vi "setting.vi"(8 "error in (no error)":errorcluster caption="错误输入（无错误）") -> (0 "error out":errorcluster caption="错误输出", 3 "设置":T1)   [LabVIEW 2018]
panel:
  in  "采集设置":T2={"Resource Name"="DAQ::1", "Input Impedance"=0, "采集通道"=2, "Trigger Level (V)"=0.5, "Coupling"=1, "Trigger Slope"=0, "Min Record Length"=40000, "Min. Sample Rate"=10000000.0, "Vertical Range (V)"=5.0, "触发通道"=2} {"触发通道" items=["ch0", "ch1", "ch2", "ch3", "ch4", "ch5", "ch6", "ch7"]; "Vertical Range (V)" format="%_3g"; "Min. Sample Rate" min=10.0 max=60000000.0 format="%#_6p"; "Trigger Slope" items=["Positive", "Negative"]; "Coupling" items=["AC"=0, "DC"=1, "HF Reject"=3, "LF Reject"=4, "AC Plus HF Reject"=1001]; "Trigger Level (V)" format="%.2f"; "采集通道" items=["ch0", "ch1", "ch2", "ch3", "ch4", "ch5", "ch6", "ch7"]; "Input Impedance" items=["1 mega ohm"=0, "50 ohms"=2]}
  in  "矩阵卡设置":cluster{"BUS":u32, "slot":u32}={"BUS"=5, "slot"=5}
  in  "取消按钮":bool
  in  "保存按钮":bool
  in  "模式一设置":T3={"M1-drive-start"=5, "M1-drive-num"=5, "M1-receive-start"=5, "M1-receive-num"=5, "M1-start-delay"=5, "M1-receive-delay"=5}
  in  "模式二设置":T4={"M2-drive-start"=5, "M2-receive-start"=5, "M2-receive-num"=5, "M2-start-delay"=5, "M2-receive-delay"=5}
  # "参数设置"
  # "数据采集"
  # "矩阵开关"
  # "模式一"
  # "模式二"
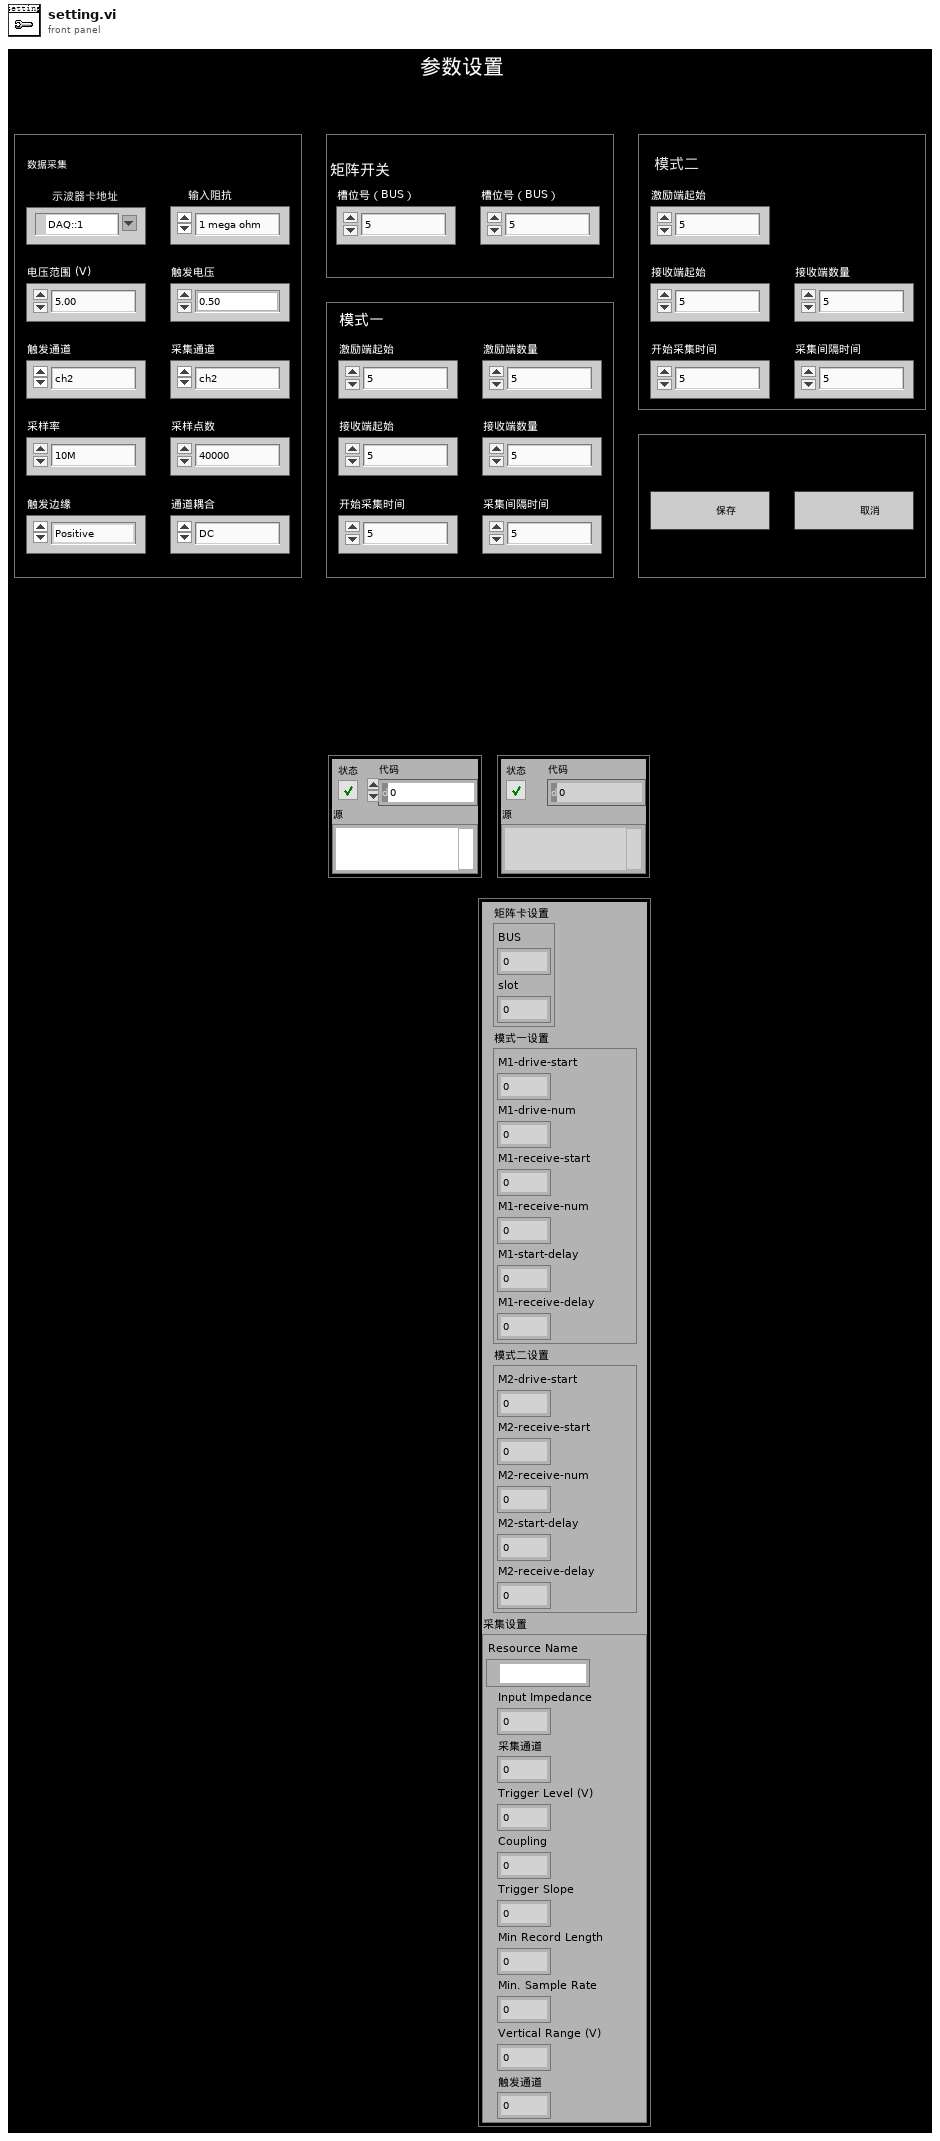
[diagram p1: front panel]
types:
  T1 = cluster{"矩阵卡设置":cluster{"BUS":u32, "slot":u32}, "模式一设置":cluster{"M1-drive-start":u32, "M1-drive-num":u32, "M1-receive-start":u32, "M1-receive-num":u32, "M1-start-delay":u32, "M1-receive-delay":u32}, "模式二设置":cluster{"M2-drive-start":u32, "M2-receive-start":u32, "M2-receive-num":u32, "M2-start-delay":u32, "M2-receive-delay":u32}, "采集设置":cluster{"Resource Name":refnum<k15>, "Input Impedance":u32, "采集通道":i32, "Trigger Level (V)":dbl, "Coupling":u16, "Trigger Slope":i32, "Min Record Length":i32, "Min. Sample Rate":dbl, "Vertical Range (V)":dbl, "触发通道":i32}}
  T2 = cluster{"Resource Name":refnum<k15>, "Input Impedance":u32, "采集通道":i32, "Trigger Level (V)":dbl, "Coupling":u16, "Trigger Slope":i32, "Min Record Length":i32, "Min. Sample Rate":dbl, "Vertical Range (V)":dbl, "触发通道":i32}
  T3 = cluster{"M1-drive-start":u32, "M1-drive-num":u32, "M1-receive-start":u32, "M1-receive-num":u32, "M1-start-delay":u32, "M1-receive-delay":u32}
  T4 = cluster{"M2-drive-start":u32, "M2-receive-start":u32, "M2-receive-num":u32, "M2-start-delay":u32, "M2-receive-delay":u32}
  T5 = typedef "LVRectTypeDef.ctl" = cluster{"Left":i16, "Top":i16, "Right":i16, "Bottom":i16}
  T6 = enum8{"Enabled", "Disabled", "Disabled and Grayed Out"}
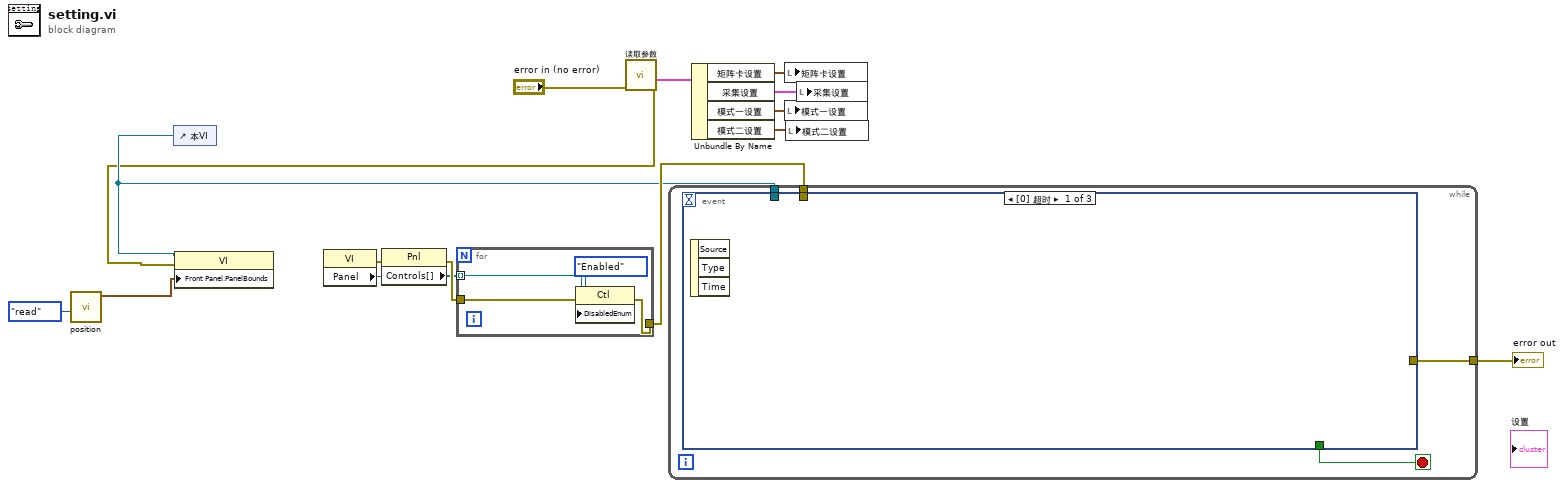
[diagram p0: block diagram]
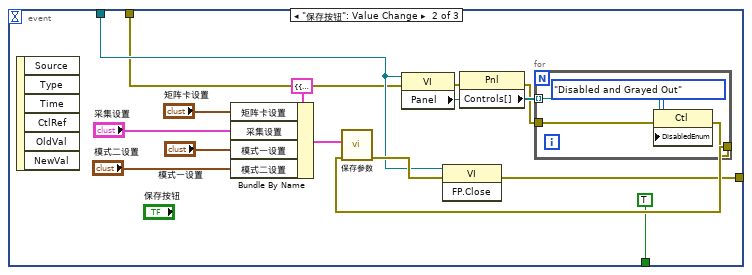
[diagram p2: hidden frame]
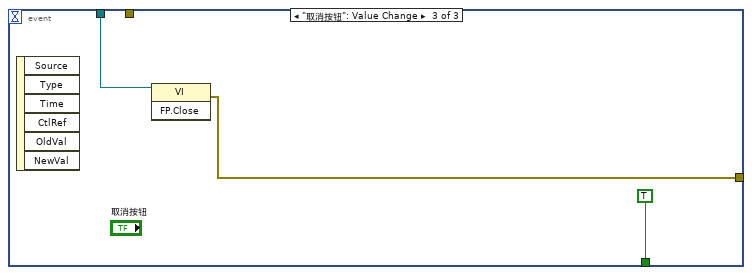
[diagram p3: hidden frame]
diagram:
  n1 = call "position.vi"("枚举"=enum16{"write", "read"}."read") -> ("前面板窗口:窗口边界 2"=w1:T5)  [unwired: 10 in]
  n2 = control-ref of="本VI"() -> (w3:refnum<vi>)
  n3 = property class="VI"() -> (error out=w8:errorcluster, "Panel"=w7:refnum<vi>)  [unwired: 2 in, 1 out]
  n4 = property class="Pnl"(reference=w7, error in=w8) -> (error out=w9:errorcluster, "Controls[]"=w6:refnum<vi>[])  [unwired: 1 out]
  n5 = for {
    tunnel: w6 -> [w20] mode=indexing
    tunnel: w9 -> [w18]
    tunnel: [w17] -> w5
    n6 = property class="Ctl"(reference=w20, error in=w18, "DisabledEnum"=T6."Enabled" ("禁用")) -> (error out=w17:errorcluster)  [unwired: 1 out]
  }
  n7 = call "读取参数.vi"("error in (no error)"="error in (no error)") -> ("error out"=w2:errorcluster, "设置"=w10:T1)  [unwired: 9 in]
  n8 = property class="VI"(reference=w3, error in=w2, "Front Panel.PanelBounds"=w1) -> ()  [unwired: 2 out]
  n9 = while {
    tunnel: w3 -> [w24]
    tunnel: w5 -> [w23]
    tunnel: [w22] -> w16
    stop <- w21 stop-if-true
    n10 = event shown="[0] 超时" {
      selector: _ -> [_ _ _]
      dyn-events: _ -> [_ _ _]
      timeout: _ -> [_ _ _]
      tunnel: w24 -> [_ w32 w47]
      tunnel: w23 -> [_ w30 _]
      tunnel: [_ w27 w45] -> w22
      tunnel: [_ TRUE TRUE] -> w21
      event Timeout {
        n11 = event-data() -> ()  [unwired: 1 in, 3 out]
      }
      event "保存按钮": Value Change {
        n12 = event-data() -> ()  [unwired: 1 in, 6 out]
        n13 = Bundle By Name(cluster=T1 {"矩阵卡设置"={"BUS"=0, "slot"=0}, "模式一设置"={"M1-drive-start"=0, "M1-drive-num"=0, "M1-receive-start"=0, "M1-receive-num"=0, "M1-start-delay"=0, "M1-receive-delay"=0}, "模式二设置"={"M2-drive-start"=0, "M2-receive-start"=0, "M2-receive-num"=0, "M2-start-delay"=0, "M2-receive-delay"=0}, "采集设置"={"Resource Name"="PXI1Slot2", "Input Impedance"=0, "采集通道"=2, "Trigger Level (V)"=0.5, "Coupling"=1, "Trigger Slope"=0, "Min Record Length"=40000, "Min. Sample Rate"=10000000.0, "Vertical Range (V)"=5.0, "触发通道"=2}} ("输入簇"), "矩阵卡设置"="矩阵卡设置", "采集设置"="采集设置", "模式一设置"="模式一设置", "模式二设置"="模式二设置") -> (w25:T1)
        n14 = property class="VI"(reference=w32, error in=w30) -> (error out=w31:errorcluster, "Panel"=w33:refnum<vi>)  [unwired: 1 out]
        n15 = property class="Pnl"(reference=w33, error in=w31) -> (error out=w29:errorcluster, "Controls[]"=w34:refnum<vi>[])  [unwired: 1 out]
        n16 = for {
          tunnel: w34 -> [w44] mode=indexing
          tunnel: w29 -> [w42]
          tunnel: [w41] -> w28
          n17 = property class="Ctl"(reference=w44, error in=w42, "DisabledEnum"=T6."Disabled and Grayed Out" ("禁用")) -> (error out=w41:errorcluster)  [unwired: 1 out]
        }
        n18 = call "保存参数.vi"("设置"=w25, "error in (no error)"=w28) -> ("error out"=w35:errorcluster)  [unwired: 7 in]
        n19 = invoke class="VI" method="FP.Close"(reference=w32, error in=w35) -> (error out=w27:errorcluster)  [unwired: 1 in, 2 out]
      }
      event "取消按钮": Value Change {
        n20 = event-data() -> ()  [unwired: 1 in, 6 out]
        n21 = invoke class="VI" method="FP.Close"(reference=w47) -> (error out=w45:errorcluster)  [unwired: 2 in, 2 out]
      }
    }
  }
  "error out" <- w16
  n22 = Unbundle By Name(w10) -> ("矩阵卡设置"=w14:cluster{"BUS":u32, "slot":u32}, "采集设置"=w13:T2, "模式一设置"=w12:T3, "模式二设置"=w11:T4)
  n23 = local write "矩阵卡设置"(w14) -> ()
  n24 = local write "模式一设置"(w12) -> ()
  n25 = local write "模式二设置"(w11) -> ()
  n26 = local write "采集设置"(w13) -> ()
